vi "Loop Async.vi"(11 "ChannelService in":refnum<class "ChannelService.lvclass">) -> ()   [LabVIEW 2020, in "Vecto.lvlib" / "ChannelService.lvclass"]
uses:
  ChannelService.lvclass
  Loop Data.ctl
  Group/Group.lvclass
  ChannelService.lvclass/ChannelService.ctl
  GroupValue/GroupValue.lvclass
  C:/Program Files (x86)/National Instruments/LabVIEW 2024/vi.lib/IlluminatedG/IG Promises/Promises/Value/Value.lvclass
  <vilib>/IlluminatedG/IG Promises/Promises/Promise/Promise.lvclass
  Group Config/Group Config.lvclass
panel:
  out "Last Created Group":string
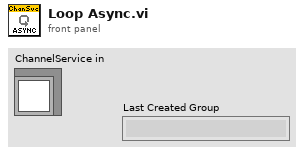
[diagram p1: front panel]
types:
  T1 = typedef "Vecto.lvlib/ChannelService.lvclass/Loop Data.ctl" = cluster{"Groups":refnum<class "Group.lvclass">[], "Channel Group Map":map{string, i32}, "Group Map":map{string, i32}}
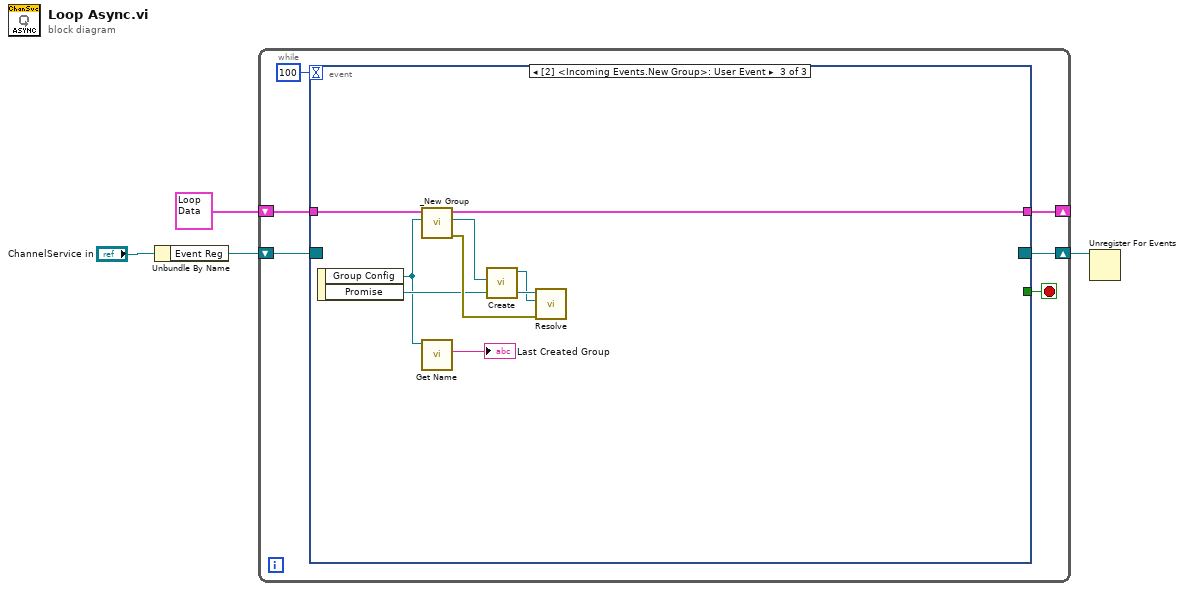
[diagram p0: block diagram]
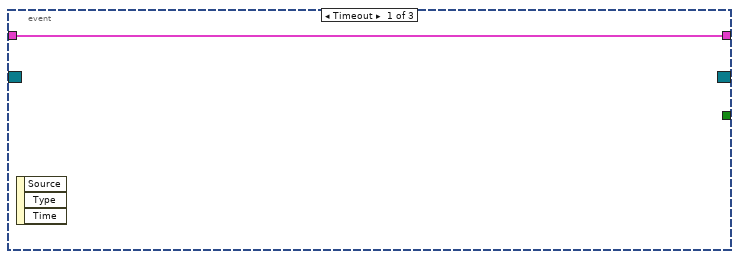
[diagram p2: hidden frame]
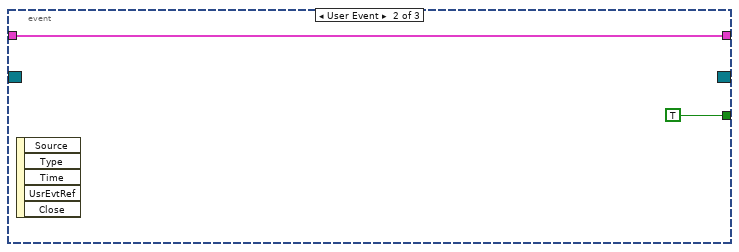
[diagram p3: hidden frame]
diagram:
  n1 = Unbundle By Name("ChannelService in") -> ("Event Reg"=w3:refnum<event-registration>)
  n2 = while {
    shift-right: [w6] -> w1
    shift-left: w3 -> [w10]
    shift-right: [w7] -> _
    shift-left: T1 {"Groups"=[], "Channel Group Map"={}, "Group Map"={}} ("Loop Data") -> [w8]
    stop <- w5 stop-if-true
    n3 = event shown="[2] <Incoming Events.New Group>: User Event" {
      selector: w10 -> [_ _ _]
      dyn-events: [_ _ _] -> w6
      timeout: 100 -> [_ _ _]
      tunnel: w8 -> [w11 w13 w20]
      tunnel: [_ TRUE _] -> w5
      tunnel: [w11 w13 w16] -> w7
      event Timeout {
        n4 = event-data() -> ()  [unwired: 1 in, 3 out]
      }
      event User Event {
        n5 = event-data() -> ()  [unwired: 1 in, 5 out]
      }
      event User Event {
        n6 = event-data() -> ("Group Config"=w15:refnum<class "Group Config.lvclass">, "Promise"=w19:refnum<class "Promise.lvclass">)  [unwired: 1 in]
        n7 = call "_New Group.vi"("Group Config"=w15, "Loop Data in"=w20) -> ("error out"=w21:errorcluster, "New Group"=w18:refnum<class "Group.lvclass">, "Loop Data"=w16:T1)  [unwired: 7 in]
        n8 = call "Get Name.vi"("Group Config in"=w15) -> ("Name"=→"Last Created Group":string)  [unwired: 8 in, 2 out]
        n9 = call "Create.vi"("Group"=w18) -> ("GroupValue out"=w17:refnum<class "GroupValue.lvclass">)  [unwired: 10 in]
        n10 = call <vilib>:"Resolve.vi"("error in (no error)"=w21, "Result"=w17, "Promise in"=w19) -> ()  [unwired: 7 in, 2 out]
      }
    }
  }
  n11 = Unregister For Events(event registration refnum=w1) -> ()  [unwired: 1 in, 1 out]
